vi "Sea-Level SWI Config Test.vi"(8 "error in (no error)":errorcluster, 10 "Configuration":T1={"BusType"=enum."PCI/ISA/PCMCIA", "Card"=0, "USB"=16, "IP"=0, "COM"=1, "Baud Rate"=enum."9600"}, 11 "Str Refnum":refnum<vi>) -> (0 "error out":errorcluster)   [LabVIEW 2011]
uses:
  TypeDefs/Sea-Level SWI Configuration.ctl
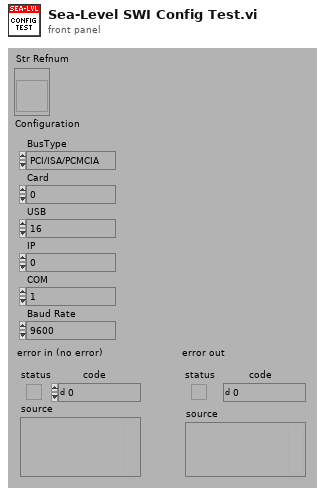
[diagram p1: front panel]
types:
  T1 = typedef "Sea-Level SWI Configuration.ctl" = cluster{"BusType":enum32{"PCI/ISA/PCMCIA", "USB", "Ethernet", "Serial"}, "Card":i32, "USB":i32, "IP":u32, "COM":i32, "Baud Rate":enum16{"300", "600", "1200", "2400", "4800", "9600"}}
  T2 = enum32{"PCI/ISA/PCMCIA", "USB", "Ethernet", "Serial"}
  T3 = typedef "Sea-Level SWI Adapter Info.ctl" = cluster{"Long Reserved 0":i32, "Long Reserved 1":i32, "Long Reserved 2":i32, "Long Reserved 3":i32, "State Capabilities":i32, "Card Number":i16, "Base IO":i16, "Port In Count":i8, "Port Out Count":i8, "Port Count":i8, "Enabled":i8, "IRQ":i16}
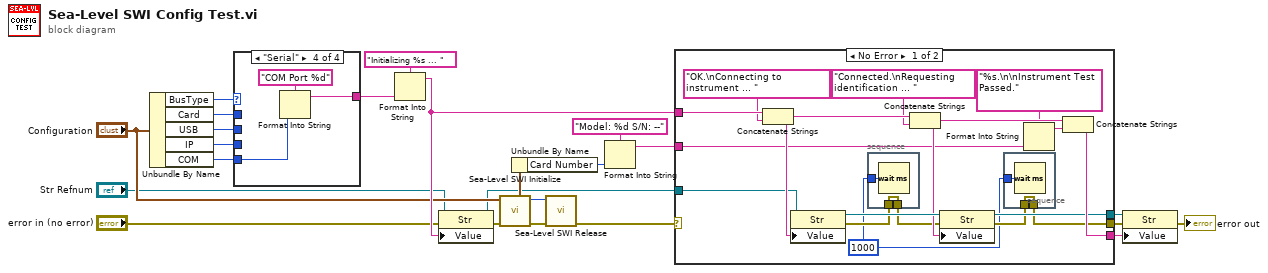
[diagram p0: block diagram]
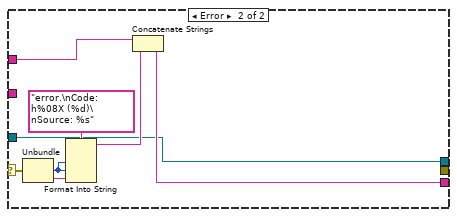
[diagram p2: hidden frame]
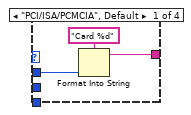
[diagram p3: hidden frame]
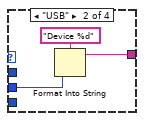
[diagram p4: hidden frame]
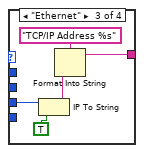
[diagram p5: hidden frame]
diagram:
  n1 = Unbundle By Name("Configuration") -> ("BusType"=w23:T2, "Card"=w22:i32, "USB"=w21:i32, "IP"=w20:u32, "COM"=w19:i32)
  n2 = case shown="\"Serial\"" w23 {
    tunnel: w22 -> [w26 _ _ _]
    tunnel: w21 -> [_ w28 _ _]
    tunnel: w20 -> [_ _ w34 _]
    tunnel: w19 -> [_ _ _ w36]
    tunnel: [w25 w29 w31 w37] -> w18
    frame "PCI/ISA/PCMCIA", Default {
      n3 = Format Into String(format string="Card %d", w26) -> (resulting string=w25:string)  [unwired: 2 in, 1 out]
    }
    frame "USB" {
      n4 = Format Into String(format string="Device %d", w28) -> (resulting string=w29:string)  [unwired: 2 in, 1 out]
    }
    frame "Ethernet" {
      n5 = IP To String(1:TRUE, 2:w34) -> (0:w33:string)
      n6 = Format Into String(format string="TCP/IP Address %s", w33) -> (resulting string=w31:string)  [unwired: 2 in, 1 out]
    }
    frame "Serial" {
      n7 = Format Into String(format string="COM Port %d", w36) -> (resulting string=w37:string)  [unwired: 2 in, 1 out]
    }
  }
  n8 = Format Into String(format string="Initializing %s ... ", w18) -> (resulting string=w17:string)  [unwired: 2 in, 1 out]
  n9 = property class="Str"(reference="Str Refnum", error in="error in (no error)", "Value"=w17) -> (reference out=w1:refnum<vi>, error out=w15:errorcluster)
  n10 = call "Sea-Level SWI Initialize.vi"("error in (no error)"=w15, "Configuration"="Configuration") -> ("error out"=w12:errorcluster, "Handle Out"=w10:i32, "Sea-Level SWI"=w9:T3)  [unwired: 7 out]
  n11 = Unbundle By Name(w9) -> ("Card Number"=w13:i16)
  n12 = call "Sea-Level SWI Release.vi"("error in (no error)"=w12, "Handle"=w10) -> ("error out"=w11:errorcluster)  [unwired: 1 in, 8 out]
  n13 = Format Into String(format string="Model: %d S/N: --" ("Return Model and Serial #"), w13) -> (resulting string=w8:string)  [unwired: 2 in, 1 out]
  n14 = case shown="No Error" w11 {
    selector: w11 -> [_ w65]
    tunnel: w17 -> [w54 w67]
    tunnel: w1 -> [w49 w60]
    tunnel: w8 -> [w46 _]
    tunnel: [w45 w61] -> w6
    tunnel: [w44 w60] -> w4
    tunnel: [w40 _] -> w3
    frame No Error {
      w39 = u32 1000 ("milliseconds to wait")
      n15 = Concatenate Strings(w54, "OK.\nConnecting to instrument ... ") -> (w52:string)
      n16 = property class="Str"(reference=w49, "Value"=w52) -> (reference out=w55:refnum<vi>, error out=w43:errorcluster)  [unwired: 1 in]
      n17 = stacked-sequence {
        tunnel: w39 -> [w59]
        tunnel: w43 -> [w58]
        tunnel: [w58] -> w42
        frame #0 {
          n18 = Wait (ms)(milliseconds to wait=w59) -> ()  [unwired: 1 out]
        }
      }
      n19 = Concatenate Strings(w52, "Connected.\nRequesting identification ... ") -> (w50:string)
      n20 = property class="Str"(reference=w55, error in=w42, "Value"=w50) -> (reference out=w44:refnum<vi>, error out=w41:errorcluster)
      n21 = stacked-sequence {
        tunnel: w39 -> [w57]
        tunnel: w41 -> [w56]
        tunnel: [w56] -> w40
        frame #0 {
          n22 = Wait (ms)(milliseconds to wait=w57) -> ()  [unwired: 1 out]
        }
      }
      n23 = Format Into String(format string="%s.\n\nInstrument Test Passed.", w46) -> (resulting string=w47:string)  [unwired: 2 in, 1 out]
      n24 = Concatenate Strings(w50, w47) -> (w45:string)
    }
    frame Error {
      n25 = Unbundle(w65) -> ("code"=w64:i32, "source"=w63:string)  [unwired: 1 out]
      n26 = Format Into String(format string="error.\nCode:  h%08X (%d)\nSource: %s", w64, w64, w63) -> (resulting string=w62:string)  [unwired: 2 in, 1 out]
      n27 = Concatenate Strings(w67, w62) -> (w61:string)
    }
  }
  n28 = property class="Str"(reference=w4, error in=w3, "Value"=w6) -> (error out=→"error out":errorcluster)  [unwired: 1 out]
